vi "VerificarVencedor.vi"(6 "Nome do Jogador":string="João", 8 "error in (no error)":errorcluster, 9 "refnum in":refnum<file>, 10 "CaracterComparacao":string="X", 11 "ArrayEntrada":string[][](array[string])=[["X", "X", "O"], ["O", "X", "O"], ["X", "O", "X"]]) -> (0 "error out":errorcluster, 1 "refnum out":refnum<file>, 2 "VenceuOuEmpatou":bool, 3 "ArraySaida":string[][](array[string])=[["X", "X", "O"], ["O", "X", "O"], ["X", "O", "X"]])   [LabVIEW 2011]
doc: "Esse VI verifica se houve vitória de algum jogador ou se houve empate (Velha)."
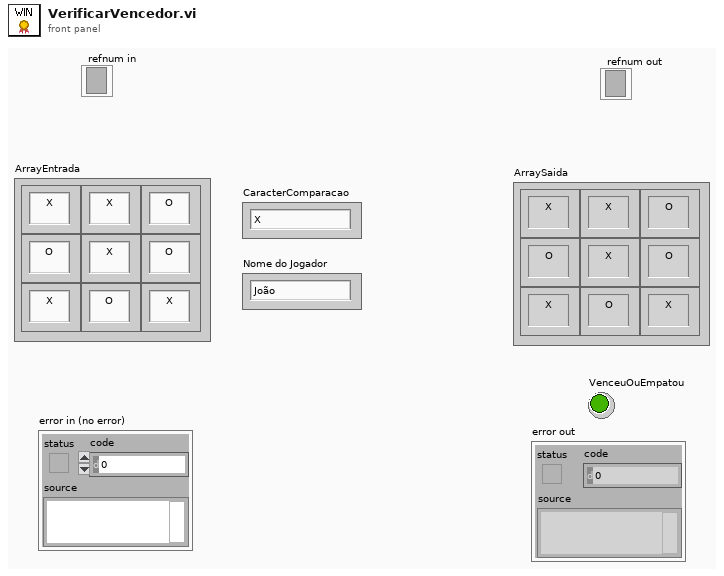
[diagram p1: front panel]
types:
  T1 = enum16{"Verifica Velha", "Verifica Vencedor", "Mensagem"}
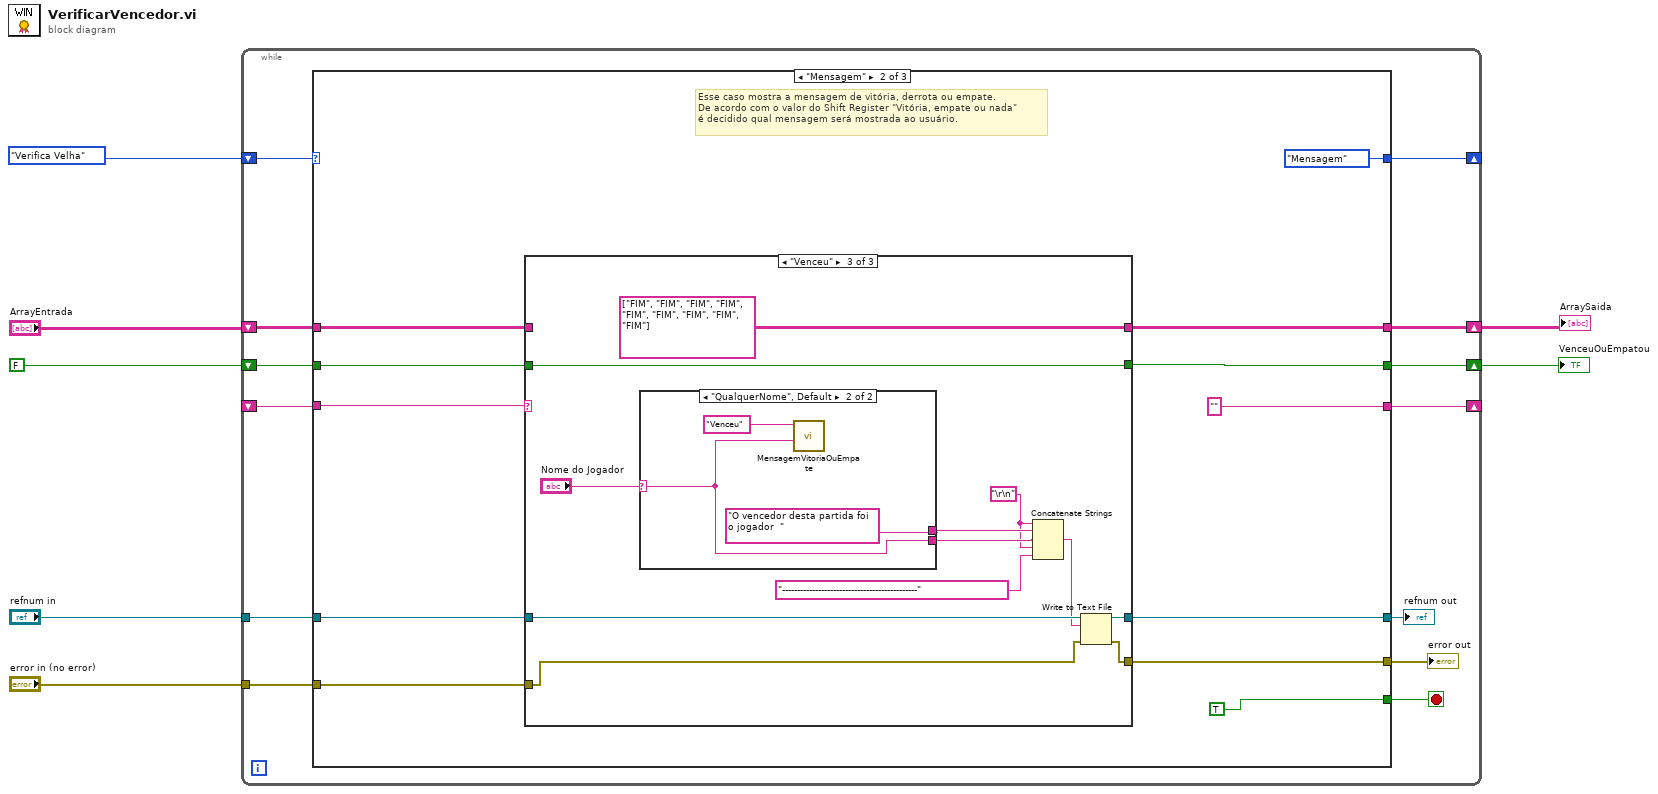
[diagram p0: block diagram]
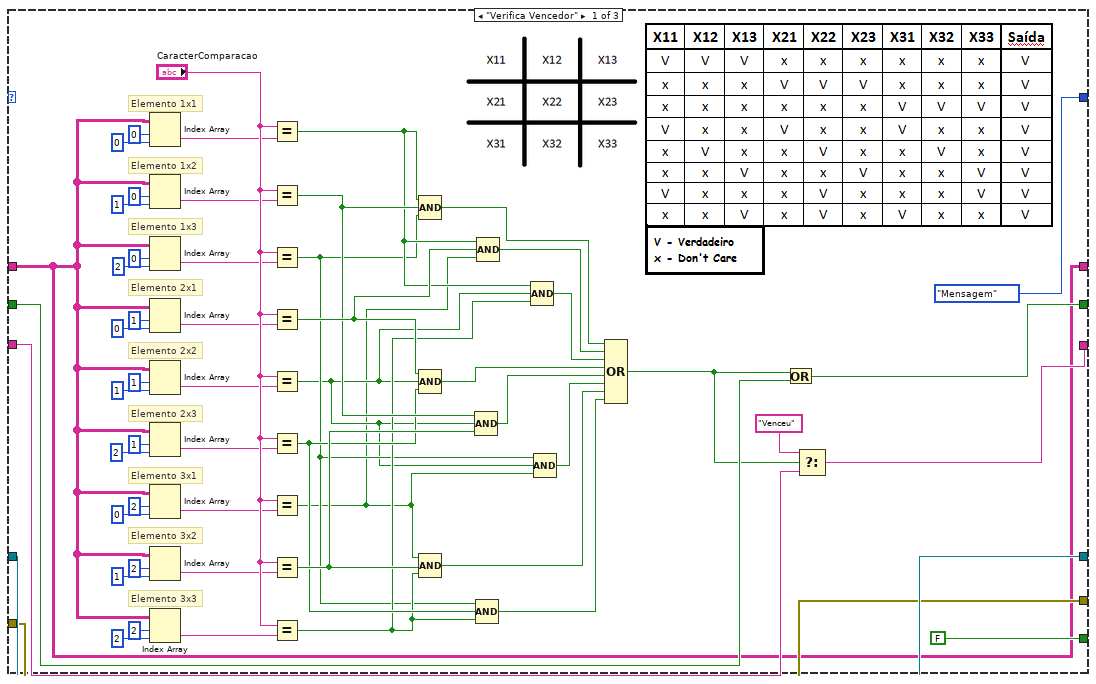
[diagram p2: hidden frame]
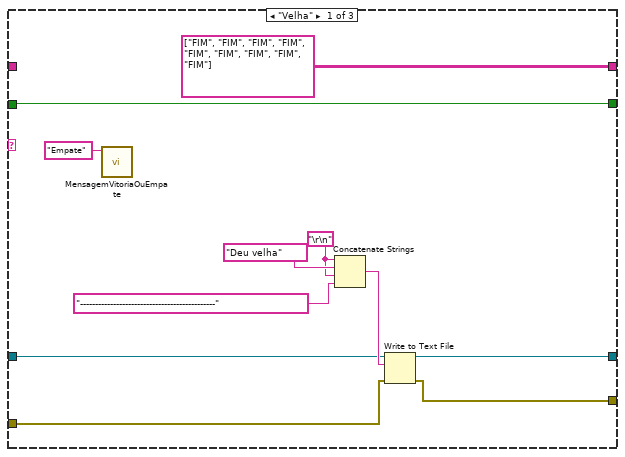
[diagram p3: hidden frame]
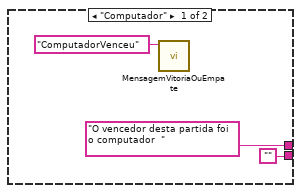
[diagram p5: hidden frame]
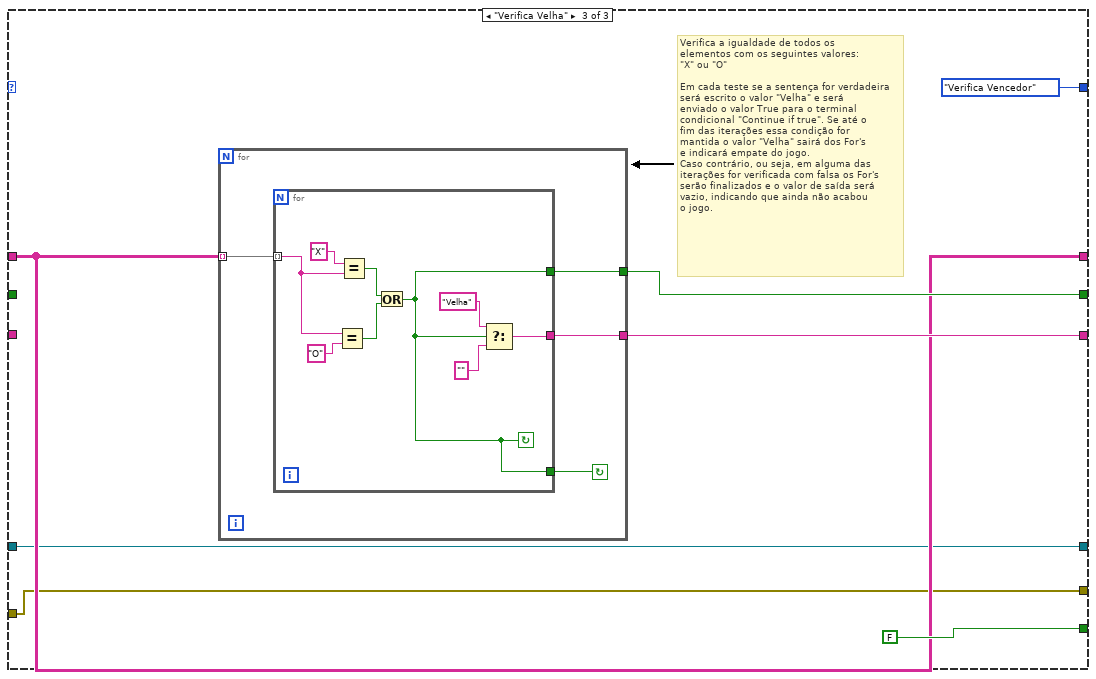
[diagram p6: hidden frame]
diagram:
  n1 = while {
    shift-right: [w20] -> _
    shift-left: T1."Verifica Velha" ("VerificaStatus") -> [w19]
    shift-right: [w17] -> _
    shift-left: _ -> [w15]
    shift-right: [w13] -> w3
    shift-left: FALSE -> [w14]
    shift-right: [w12] -> w5
    shift-left: "ArrayEntrada" -> [w16]
    tunnel: "refnum in" -> [w11]
    tunnel: "error in (no error)" -> [w9]
    stop <- w18 stop-if-true
    n2 = case shown="\"Mensagem\"" w19 {
      tunnel: [T1."Mensagem" ("VerificaStatus") T1."Mensagem" ("VerificaStatus") T1."Verifica Vencedor" ("VerificaStatus")] -> w20
      tunnel: [FALSE TRUE FALSE] -> w18
      tunnel: [w23 "" ("f") w126] -> w17
      tunnel: w16 -> [w21 w84 w124]
      tunnel: w15 -> [w30 w88 _]
      tunnel: [w26 w79 w125] -> w13
      tunnel: w14 -> [w28 w80 _]
      tunnel: [w21 w83 w124] -> w12
      tunnel: w11 -> [w29 w82 w123]
      tunnel: [w29 w81 w123] -> w10
      tunnel: w9 -> [w25 w78 w122]
      tunnel: [w25 w77 w122] -> w8
      frame "Verifica Vencedor" {
        # "Elemento 3x3"
        # "Elemento 3x2"
        # "Elemento 3x1"
        # "Elemento 2x3"
        # "Elemento 2x2"
        # "Elemento 2x1"
        # "Elemento 1x3"
        # "Elemento 1x2"
        # "Elemento 1x1"
        n3 = Index Array(array=w21, index (row)=0, index (col)=0 ("disabled index (col)")) -> (element=w39:string)
        n4 = Index Array(array=w21, index (row)=0, index (col)=1 ("disabled index (col)")) -> (element=w38:string)
        n5 = Index Array(array=w21, index (row)=0, index (col)=2 ("disabled index (col)")) -> (element=w37:string)
        n6 = Index Array(array=w21, index (row)=1, index (col)=0 ("disabled index (col)")) -> (element=w36:string)
        n7 = Index Array(array=w21, index (row)=1, index (col)=1 ("disabled index (col)")) -> (element=w35:string)
        n8 = Index Array(array=w21, index (row)=1, index (col)=2 ("disabled index (col)")) -> (element=w34:string)
        n9 = Index Array(array=w21, index (row)=2, index (col)=0 ("disabled index (col)")) -> (element=w33:string)
        n10 = Index Array(array=w21, index (row)=2, index (col)=1 ("disabled index (col)")) -> (element=w32:string)
        n11 = Index Array(array=w21, index (row)=2, index (col)=2 ("disabled index (col)")) -> (element=w31:string)
        n12 = Equal?(x="CaracterComparacao", y=w39) -> (x = y?=w52:bool)
        n13 = Equal?(x="CaracterComparacao", y=w38) -> (x = y?=w55:bool)
        n14 = Equal?(x="CaracterComparacao", y=w37) -> (x = y?=w50:bool)
        n15 = Equal?(x="CaracterComparacao", y=w36) -> (x = y?=w56:bool)
        n16 = Equal?(x="CaracterComparacao", y=w35) -> (x = y?=w49:bool)
        n17 = Equal?(x="CaracterComparacao", y=w34) -> (x = y?=w53:bool)
        n18 = Equal?(x="CaracterComparacao", y=w33) -> (x = y?=w48:bool)
        n19 = Equal?(x="CaracterComparacao", y=w32) -> (x = y?=w54:bool)
        n20 = Equal?(x="CaracterComparacao", y=w31) -> (x = y?=w51:bool)
        n21 = Compound Arithmetic op=AND(w52, w55, w50) -> (w24:bool)
        n22 = Compound Arithmetic op=AND(w56, w49, w53) -> (w45:bool)
        n23 = Compound Arithmetic op=AND(w48, w54, w51) -> (w42:bool)
        n24 = Compound Arithmetic op=AND(w55, w49, w54) -> (w44:bool)
        n25 = Compound Arithmetic op=AND(w50, w53, w51) -> (w41:bool)
        n26 = Compound Arithmetic op=AND(w52, w56, w48) -> (w47:bool)
        n27 = Compound Arithmetic op=AND(w52, w49, w51) -> (w46:bool)
        n28 = Compound Arithmetic op=AND(w50, w49, w48) -> (w43:bool)
        n29 = Compound Arithmetic op=OR(w24, w47, w46, w45, w44, w43, w42, w41) -> (w27:bool)
        n30 = Or(x=w27, y=w28) -> (x .or. y?=w26:bool)
        n31 = Select(t="Venceu", s=w27, f=w30) -> (s? t:f=w23:string)
      }
      frame "Mensagem" {
        # "Esse caso mostra a mensagem de vitória, derrota ou empate.\nDe acordo com o valor do Shift Register \"Vitória, empate ou nada\"\né decidido qual mensagem será mostrada ao usuário."
        n32 = case shown="\"Venceu\"" w88 {
          tunnel: [string[][] [["FIM", "FIM", "FIM"], ["FIM", "FIM", "FIM"], ["FIM", "FIM", "FIM"]] ("ArrayConstante") w102 string[][] [["FIM", "FIM", "FIM"], ["FIM", "FIM", "FIM"], ["FIM", "FIM", "FIM"]] ("ArrayConstante")] -> w83
          tunnel: w84 -> [_ w102 _]
          tunnel: w82 -> [w92 w103 w114]
          tunnel: [w93 w103 w113] -> w81
          tunnel: w80 -> [w91 w101 w106]
          tunnel: [w91 w101 w106] -> w79
          tunnel: w78 -> [w90 w100 w105]
          tunnel: [w89 w100 w104] -> w77
          frame "Velha" {
            w95 = "\r\n"
            n33 = call "MensagemVitoriaOuEmpate.vi"("Selecao"="Empate") -> ()  [unwired: 11 in]
            n34 = Concatenate Strings(w95, "Deu velha", w95, "---------------------------------------------" ("string")) -> (w97:string)
            n35 = Write to Text File(file (use dialog)=w92, text=w97, error in=w90) -> (refnum out=w93:refnum<file>, error out=w89:errorcluster)  [unwired: 1 in, 1 out]
          }
          frame "Nada", Default {
          }
          frame "Venceu" {
            w108 = "\r\n"
            n36 = case shown="\"QualquerNome\", Default" "Nome do Jogador" {
              selector: "Nome do Jogador" -> [_ w119]
              tunnel: ["O vencedor desta partida foi o computador  " "O vencedor desta partida foi o jogador  "] -> w110
              tunnel: ["" w119] -> w109
              frame "Computador" {
                n37 = call "MensagemVitoriaOuEmpate.vi"("Selecao"="ComputadorVenceu") -> ()  [unwired: 11 in]
              }
              frame "QualquerNome", Default {
                n38 = call "MensagemVitoriaOuEmpate.vi"("Nome do Jogador"=w119, "Selecao"="Venceu") -> ()  [unwired: 10 in]
              }
            }
            n39 = Concatenate Strings(w108, w110, w109, w108, "---------------------------------------------" ("string")) -> (w111:string)
            n40 = Write to Text File(file (use dialog)=w114, text=w111, error in=w105) -> (refnum out=w113:refnum<file>, error out=w104:errorcluster)  [unwired: 1 in, 1 out]
          }
        }
      }
      frame "Verifica Velha" {
        # "Verifica a igualdade de todos os \nelementos com os seguintes valores:\n\"X\" ou \"O\"\n\nEm cada teste se a sentença for verdadeira\nserá escrito o valor \"Velha\" e será \nenviado o valor True para o terminal\ncondicional \"Continue if true\". Se até o \nfim das iterações essa condição for \nmantida o valor \"Velha\" sairá dos For's \ne indicará empate do jogo.\nCaso contrário, ou seja, em alguma das \niterações for verificada com falsa os For's \nserão finalizados e o valor de saída será \nvazio, indicando que ainda não acabou \no jogo."
        n41 = for {
          tunnel: [w132] -> w126
          tunnel: w124 -> [w130] mode=indexing
          tunnel: [w129] -> w125
          stop <- w131 continue-if-true
          n42 = for {
            tunnel: [w135] -> w132
            tunnel: [w133] -> w131
            tunnel: w130 -> [w134] mode=indexing
            tunnel: [w133] -> w129
            stop <- w133 continue-if-true
            n43 = Equal?(x=w134, y="O") -> (x = y?=w138:bool)
            n44 = Equal?(x="X", y=w134) -> (x = y?=w139:bool)
            n45 = Or(x=w139, y=w138) -> (x .or. y?=w133:bool)
            n46 = Select(t="Velha", s=w133, f="") -> (s? t:f=w135:string)
          }
        }
      }
    }
    "refnum out" <- w10
    "error out" <- w8
  }
  "ArraySaida" <- w5
  "VenceuOuEmpatou" <- w3
